vi "SubVI Tester.vi"() -> ()   [LabVIEW 2012]
panel:
  out "警告文本":string="无警告"
  out "警告？":bool
  out "温度计":dbl(slide) scale=0.0..100.0
  in  "最低温度":dbl=10.0
  in  "最高温度":dbl=30.0
  in  "停止":bool
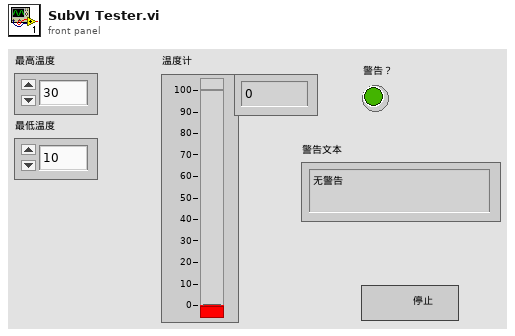
[diagram p1: front panel]
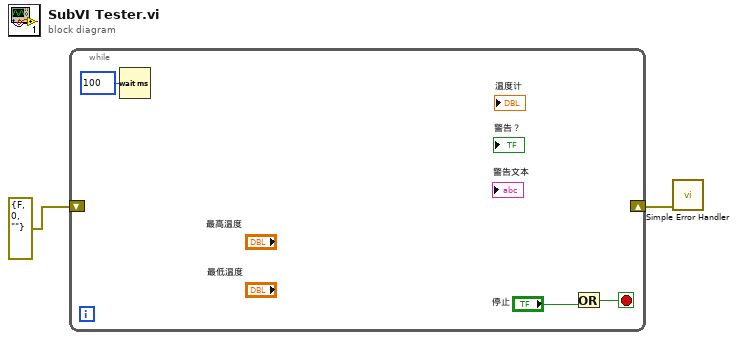
[diagram p0: block diagram]
diagram:
  n1 = while {
    shift-right: [_] -> w2
    shift-left: cluster{"状态":bool, "代码":i32, "源":string} {"状态"=FALSE, "代码"=0, "源"=""} ("错误输入") -> [_]
    stop <- w3 stop-if-true
    n2 = Wait (ms) ("等待(ms)")(milliseconds to wait=u32 100 ("等待时间（毫秒）")) -> ()  [unwired: 1 out]
    n3 = Or ("或")(y="停止") -> (x .or. y?=w3:bool)  [unwired: 1 in]
  }
  n4 = call <vilib>:"Simple Error Handler.vi"("error in (no error)"=w2) -> ()  [unwired: 4 in, 5 out]
